vi "ATSpectrograph_getEvent_lsState.vi"(8 "error in (no error)":errorcluster, 11 "logevent_lsState_Ctl":T1) -> (0 "error out":errorcluster, 2 "function return":i32, 3 "logevent_lsState_Ctl out":T1)   [LabVIEW 2016, in "SALLV_ATSpectrograph.lvlib"]
doc: "int ATSpectrograph_shm_getEvent_lsStateLV(ATSpectrograph_logevent_lsStateLV *logevent_lsState_Ctl );"
uses:
  SALLV_ATSpectrograph.lvlib
  DataTypes/logevent_lsState.ctl
  SALLV_ATSpectrograph.so
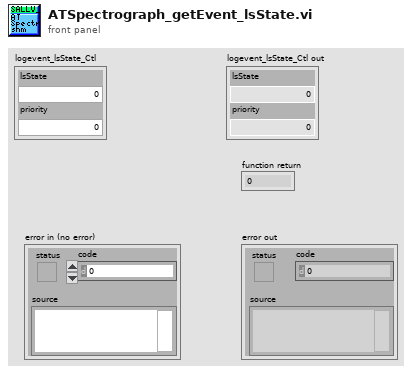
[diagram p1: front panel]
types:
  T1 = typedef "SALLV_ATSpectrograph.lvlib/logevent_lsState.ctl" = cluster{"lsState":i32, "priority":i32}
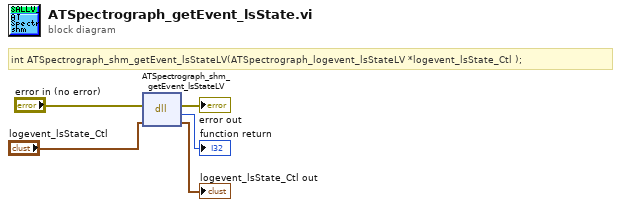
[diagram p0: block diagram]
diagram:
  # "int ATSpectrograph_shm_getEvent_lsStateLV(ATSpectrograph_logevent_lsStateLV *logevent_lsState_Ctl );"
  n1 = dll-call lib="home/harini/tcs/SALLV_ATSpectrograph/SALLV_ATSpectrograph.*" fn="ATSpectrograph_shm_getEvent_lsStateLV"(error in="error in (no error)", "logevent_lsState_Ctl"="logevent_lsState_Ctl") -> (error out=→"error out":errorcluster, →"function return":i32, "logevent_lsState_Ctl"=→"logevent_lsState_Ctl out":T1)  [unwired: 2 in, 1 out]
